vi "ExSubOpen2CamPTG.vi"(5 "Temperature":dbl format="%.2f", 6 "Temperature 2":dbl format="%.2f", 7 "error in (no error)":errorcluster) -> (0 "Camera Handle":u32, 1 "Pulser Handle":u32, 2 "Camera Handle 2":u32, 3 "Pulser Handle 2":u32, 4 "error out":errorcluster)   [LabVIEW 2010]
panel:
  # "ExSubOpen2CamPTG:\nThis sub vi opens two cameras\nand PTG systems. It sets the \ntemperature also."
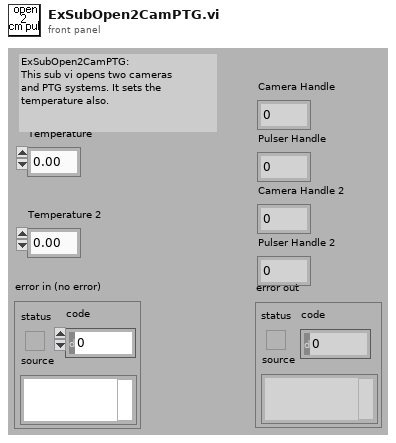
[diagram p1: front panel]
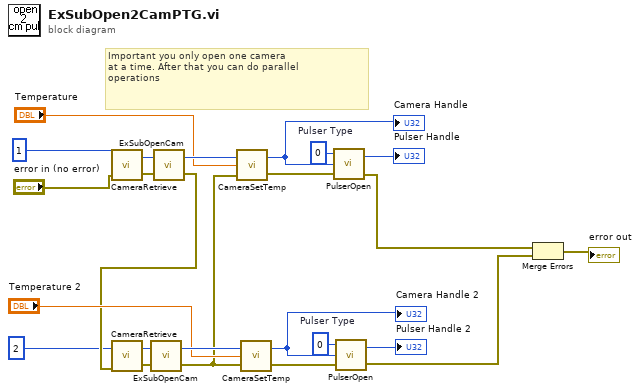
[diagram p0: block diagram]
diagram:
  w14 = u32 0  # Pulser Type
  w23 = u32 0  # Pulser Type
  # "Important you only open one camera \nat a time. After that you can do parallel \noperations"
  n1 = call <userlib>:"CameraRetrieve.vi"("error in"="error in (no error)", "Camera Index"=1) -> ("error out"=w21:errorcluster, "Device ID"=w20:u32)
  n2 = call "ExSubOpenCam.vi"("error in (no error)"=w21, "Camera Device ID"=w20) -> ("error out"=w7:errorcluster, "Camera Handle"=w19:u32)
  n3 = call <userlib>:"CameraRetrieve.vi"("error in"=w7, "Camera Index"=2) -> ("error out"=w13:errorcluster, "Device ID"=w12:u32)
  n4 = call "ExSubOpenCam.vi"("error in (no error)"=w13, "Camera Device ID"=w12) -> ("error out"=w4:errorcluster, "Camera Handle"=w11:u32)
  n5 = call <userlib>:"CameraSetTemp.vi"("error in (no error)"=w4, "Temperature"="Temperature", "Camera Handle"=w19) -> ("error out"=w17:errorcluster, "Camera Handle"=w18:u32)
  "Camera Handle" <- w18
  n6 = call <userlib>:"CameraSetTemp.vi"("error in (no error)"=w4, "Temperature"="Temperature 2", "Camera Handle"=w11) -> ("error out"=w9:errorcluster, "Camera Handle"=w10:u32)
  "Camera Handle 2" <- w10
  n7 = call <userlib>:"PulserOpen.vi"("error in"=w17, "Camera Handle"=w18, "Pulser Type"=w23) -> ("error out"=w2:errorcluster, "Pulser Handle"=→"Pulser Handle":u32)
  n8 = call <userlib>:"PulserOpen.vi"("error in"=w9, "Camera Handle"=w10, "Pulser Type"=w14) -> ("error out"=w1:errorcluster, "Pulser Handle"=→"Pulser Handle 2":u32)
  n9 = Merge Errors(w2, w1) -> (→"error out":errorcluster)
